vi "Create_Comparator_message.vi"(0 "Time":dbl, 1 "GPS timestamp":T1, 2 "Database":u8, 5 "Array":u8[](array[numeric]), 7 "Device identifier":u8, 9 "Get all elements?":bool=TRUE, 11 "Status/Errors in":refnum<vi>, 12 "Master?":bool=TRUE, 14 "Queues":T2) -> (15 "Status/Errors out":refnum<vi>)   [LabVIEW 2010]
uses:
  Controls/Queues.ctl
  Controls/One_Second.ctl
  Controls/GPS_Timestamp.ctl
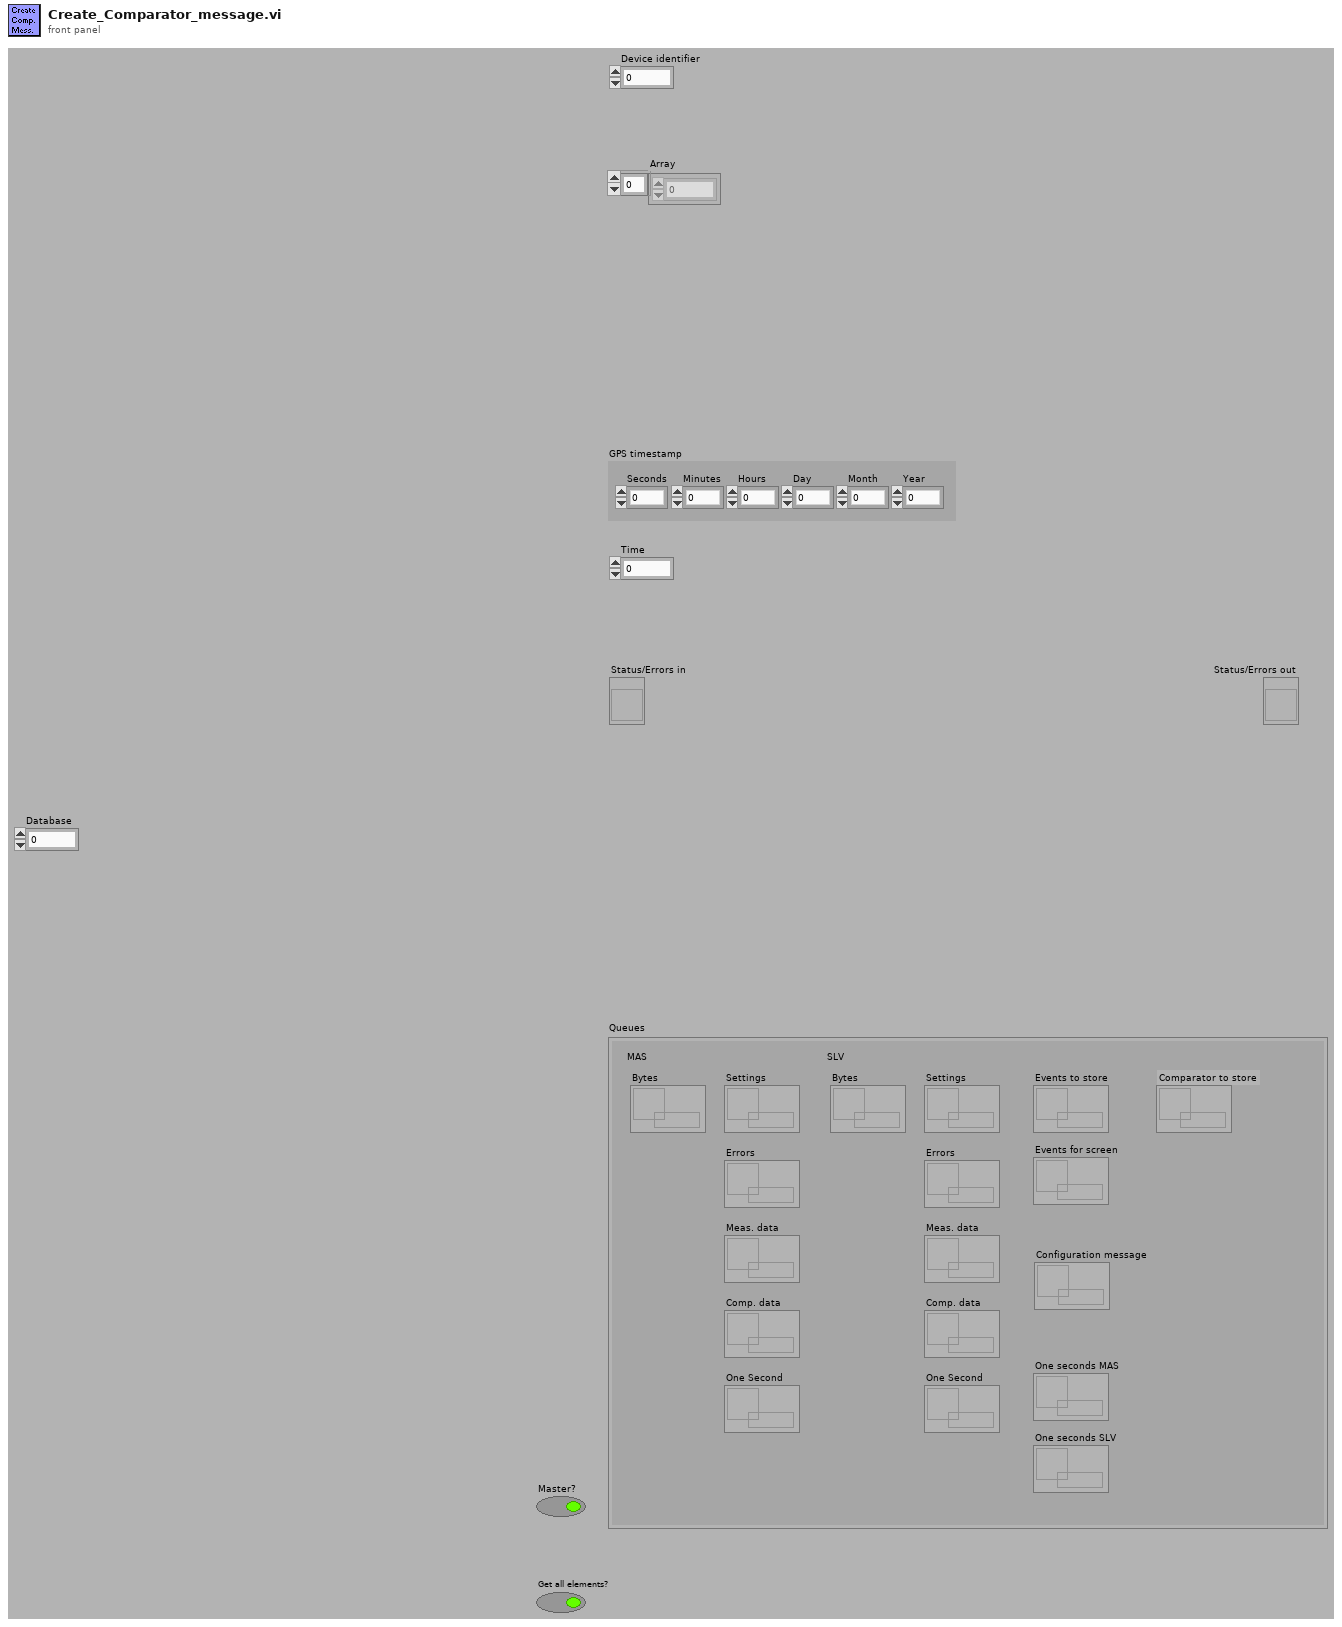
[diagram p1: front panel]
types:
  T1 = typedef "GPS_Timestamp.ctl" = cluster{"Seconds":u8, "Minutes":u8, "Hours":u8, "Day":u8, "Month":u8, "Year":u16}
  T2 = typedef "Queues.ctl" = cluster{"MAS":cluster{"Bytes":refnum<queue>, "Settings":refnum<queue>, "Errors":refnum<queue>, "Meas. data":refnum<queue>, "One Second":refnum<queue>, "Comp. data":refnum<queue>}, "SLV":cluster{"Bytes":refnum<queue>, "Settings":refnum<queue>, "Errors":refnum<queue>, "Meas. data":refnum<queue>, "One Second":refnum<queue>, "Comp. data":refnum<queue>}, "Events to store":refnum<queue>, "Events for screen":refnum<queue>, "One seconds MAS":refnum<queue>, "One seconds SLV":refnum<queue>, "Configuration message":refnum<queue>, "Comparator to store":refnum<queue>}
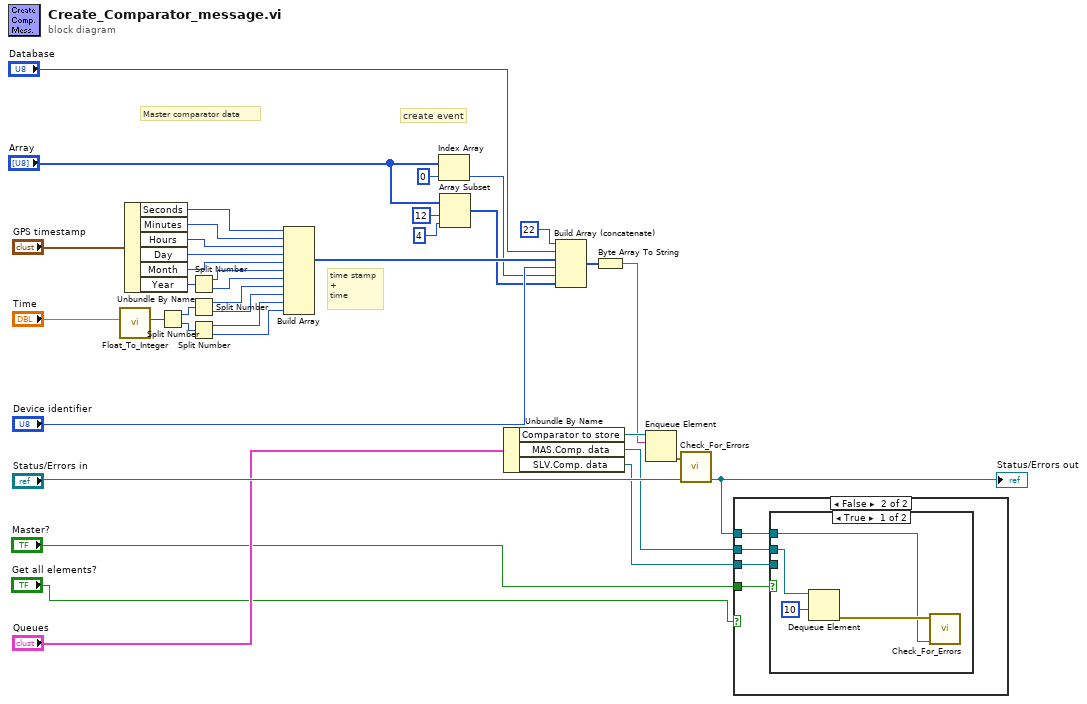
[diagram p0: block diagram]
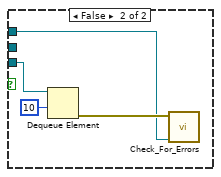
[diagram p3: hidden frame]
diagram:
  # "Master comparator data"
  # "time stamp\n+\ntime"
  # "create event"
  n1 = call "Float_To_Integer.vi"("Double"="Time") -> ("32bit integer"=w18:i32)  [unwired: 10 out]
  n2 = Unbundle By Name("GPS timestamp") -> ("Seconds"=w37:u8, "Minutes"=w36:u8, "Hours"=w35:u8, "Day"=w34:u8, "Month"=w33:u8, "Year"=w38:u16)
  n3 = Split Number(x=w18) -> (hi(x)=w29:u16, lo(x)=w30:u16)
  n4 = Split Number(x=w38) -> (hi(x)=w32:u8, lo(x)=w31:u8)
  n5 = Split Number(x=w29) -> (hi(x)=w28:u8, lo(x)=w27:u8)
  n6 = Split Number(x=w30) -> (hi(x)=w26:u8, lo(x)=w25:u8)
  n7 = Build Array(w37, w36, w35, w34, w33, w32, w31, w28, w27, w26, w25) -> (w16:u8[])
  n8 = Index Array(array="Array", index=0) -> (element=w12:u8)
  n9 = Array Subset(array="Array", index=12, length=4) -> (w8:u8[])
  n10 = Unbundle By Name("Queues") -> ("Comparator to store"=w23:refnum<queue>, "MAS.Comp. data"=w5:refnum<queue>, "SLV.Comp. data"=w6:refnum<queue>)
  n11 = Build Array (concatenate)(u8 22 ("index"), "Database", w16, "Device identifier", w12, w8) -> (w15:u8[])
  n12 = Byte Array To String(unsigned byte array=w15) -> (string=w14:string)
  n13 = Enqueue Element(queue=w23, element=w14) -> (error out=w24:errorcluster)  [unwired: 1 in, 3 out]
  n14 = call "Check_For_Errors.vi"("Status/Errors in"="Status/Errors in", "error in"=w24) -> ("Status/Errors out"=w4:refnum<vi>)  [unwired: 9 out]
  "Status/Errors out" <- w4
  n15 = case shown="False" "Get all elements?" {
    tunnel: "Master?" -> [_ w42]
    tunnel: w6 -> [_ w41]
    tunnel: w5 -> [_ w40]
    tunnel: w4 -> [_ w39]
    frame True {
    }
    frame False {
      n16 = case shown="True" w42 {
        tunnel: w41 -> [_ w48]
        tunnel: w40 -> [w46 _]
        tunnel: w39 -> [w43 w47]
        frame True {
          n17 = Dequeue Element(queue=w46, timeout in ms (-1)=10) -> (error out=w45:errorcluster)  [unwired: 1 in, 3 out]
          n18 = call "Check_For_Errors.vi"("Status/Errors in"=w43, "error in"=w45) -> ()  [unwired: 10 out]
        }
        frame False {
          n19 = Dequeue Element(queue=w48, timeout in ms (-1)=10) -> (error out=w49:errorcluster)  [unwired: 1 in, 3 out]
          n20 = call "Check_For_Errors.vi"("Status/Errors in"=w47, "error in"=w49) -> ()  [unwired: 10 out]
        }
      }
    }
  }
